vi "check_generate_new_puff_array.vi"(0 "Input References Cluster":T2, 1 "Input values cluster":T1) -> (2 "Output References Cluster":T2, 3 "Need new puff array?":bool, 4 "Output values cluster":T1)   [LabVIEW 2010]
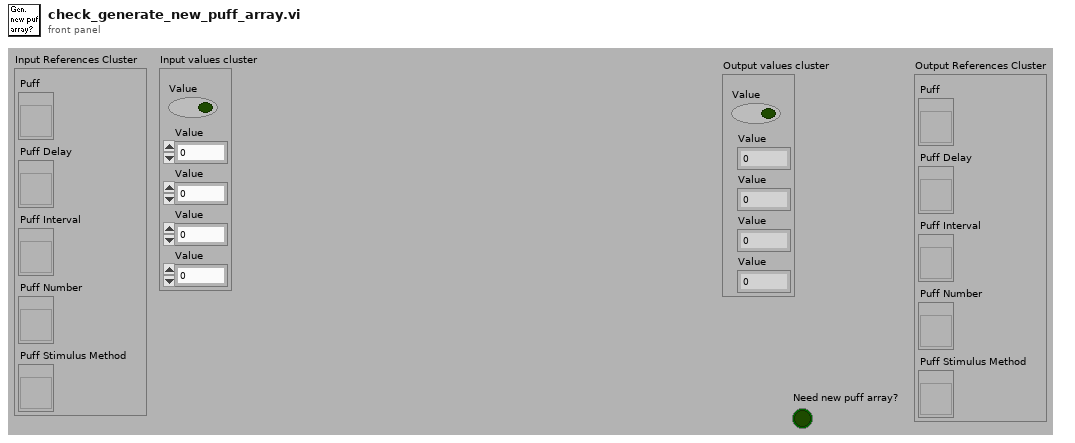
[diagram p1: front panel]
types:
  T1 = cluster{"Value":bool, "Value":dbl, "Value":dbl, "Value":dbl, "Value":u16}
  T2 = cluster{"Puff":refnum<vi>, "Puff Delay":refnum<vi>, "Puff Interval":refnum<vi>, "Puff Number":refnum<vi>, "Puff Stimulus Method":refnum<vi>}
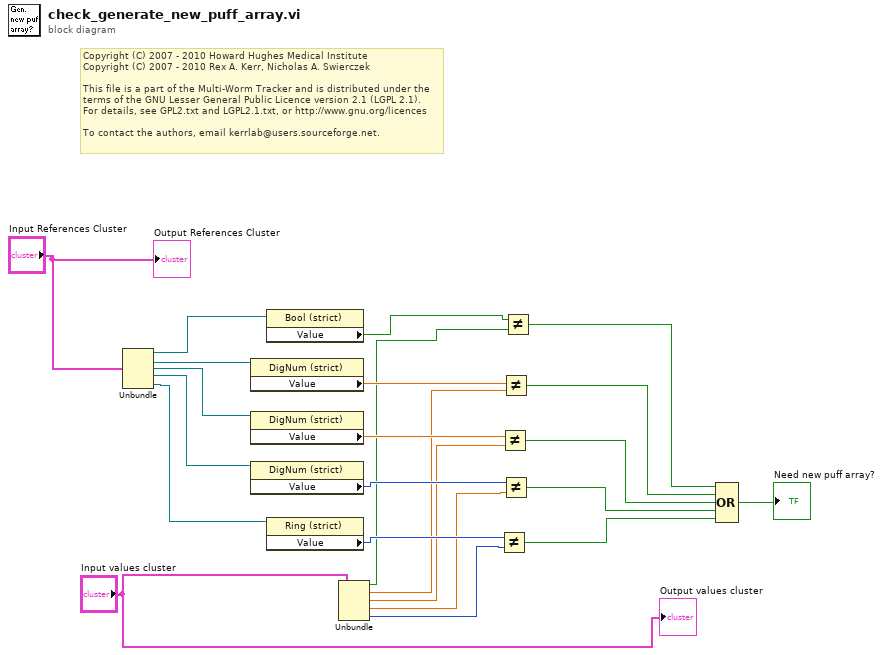
[diagram p0: block diagram]
diagram:
  # "Copyright (C) 2007 - 2010 Howard Hughes Medical Institute\nCopyright (C) 2007 - 2010 Rex A. Kerr, Nicholas A. Swierczek\n \nThis file is a part of the Multi-Worm Tracker and is distributed under the\nterms of the GNU Lesser General Public Licence version 2.1 (LGPL 2.1).\nFor details, see GPL2.txt and LGPL2.1.txt, or http://www.gnu.org/licences\n \nTo contact the authors, email kerrlab@users.sourceforge.net."
  n1 = Unbundle("Input References Cluster") -> ("Puff"=w23:refnum<vi>, "Puff Delay"=w22:refnum<vi>, "Puff Interval"=w21:refnum<vi>, "Puff Number"=w20:refnum<vi>, "Puff Stimulus Method"=w19:refnum<vi>)
  n2 = property class="DigNum (strict)"(reference=w22) -> ("Value"=w17:dbl)  [unwired: 1 in, 2 out]
  n3 = property class="DigNum (strict)"(reference=w21) -> ("Value"=w16:dbl)  [unwired: 1 in, 2 out]
  n4 = property class="DigNum (strict)"(reference=w20) -> ("Value"=w15:i32)  [unwired: 1 in, 2 out]
  n5 = property class="Bool (strict)"(reference=w23) -> ("Value"=w18:bool)  [unwired: 1 in, 2 out]
  n6 = property class="Ring (strict)"(reference=w19) -> ("Value"=w14:u16)  [unwired: 1 in, 2 out]
  n7 = Unbundle("Input values cluster") -> ("Value"=w13:bool, "Value"=w12:dbl, "Value"=w11:dbl, "Value"=w10:dbl, "Value"=w9:u16)
  n8 = Not Equal?(x=w14, y=w9) -> (x != y?=w4:bool)
  n9 = Not Equal?(x=w16, y=w11) -> (x != y?=w6:bool)
  n10 = Not Equal?(x=w17, y=w12) -> (x != y?=w7:bool)
  n11 = Not Equal?(x=w15, y=w10) -> (x != y?=w5:bool)
  n12 = Not Equal?(x=w18, y=w13) -> (x != y?=w8:bool)
  n13 = Compound Arithmetic op=OR(w8, w7, w6, w5, w4) -> (→"Need new puff array?":bool)
  "Output References Cluster" <- "Input References Cluster"
  "Output values cluster" <- "Input values cluster"
